vi "main.vi"() -> ()   [LabVIEW 2020]
panel:
  in  "대기 시간 (ms)":u32
  out "Waveform Graph":waveform(dbl)[](graph)
  in  "path":path
  in  "Channel":dbl
  in  "Sample value":dbl
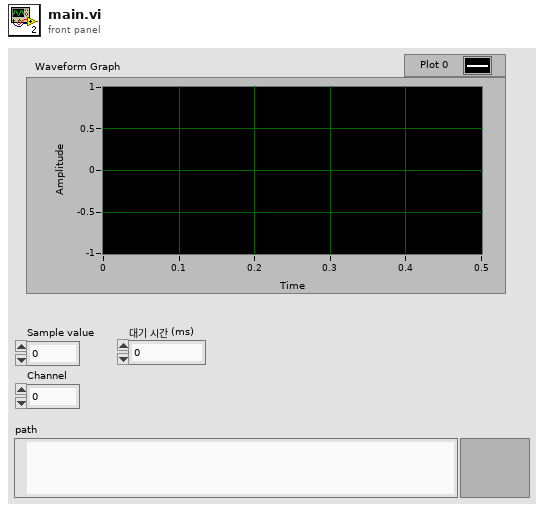
[diagram p1: front panel]
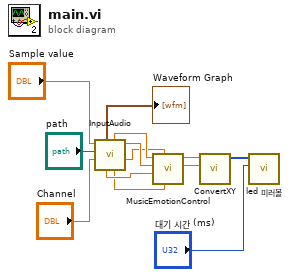
[diagram p0: block diagram]
diagram:
  n1 = call "InputAudio.vi"("Channel"="Channel", "path"="path", "Sample value"="Sample value") -> ("Centroid"=w7:dbl, "RMS"=w8:dbl, "Roll up"=w5:dbl, "BPM"=w9:dbl, "Zero Crossing"=w6:dbl, "Waveform Graph"=→"Waveform Graph":waveform(dbl)[])  [unwired: 2 in, 1 out]
  n2 = call "MusicEmotionControl.vi"("Roll off"=w5, "Centroid"=w7, "Zero Crossing"=w6, "RMS"=w8, "BPM"=w9) -> ("흥분도"=w3:dbl, "행복도"=w4:dbl)  [unwired: 4 in, 1 out]
  n3 = call "ConvertXY.vi"("흥분도(Y)"=w3, "행복도(X)"=w4) -> ("Color"=w1:u32[])  [unwired: 9 in]
  n4 = call "led 미러볼.vi"("대기 시간 (ms)"="대기 시간 (ms)", "배열"=w1) -> ()  [unwired: 9 in, 1 out]
